vi "Send Request.vi"(8 "error in (no error)":errorcluster, 11 "MJPEG Reader in":refnum<class "MJPEG Reader.lvclass">) -> (0 "error out":errorcluster, 3 "MJPEG Reader out":refnum<class "MJPEG Reader.lvclass">)   [LabVIEW 2015, in "MJPEG Reader.lvclass"]
uses:
  MJPEG Reader.lvclass
  MJPEG Reader.lvclass/MJPEG Reader.ctl
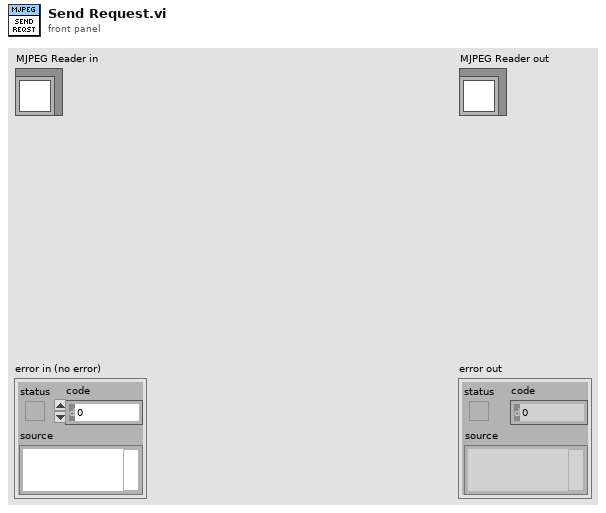
[diagram p1: front panel]
types:
  T1 = enum16{"Standard", "Buffered", "CRLF", "Immediate"}
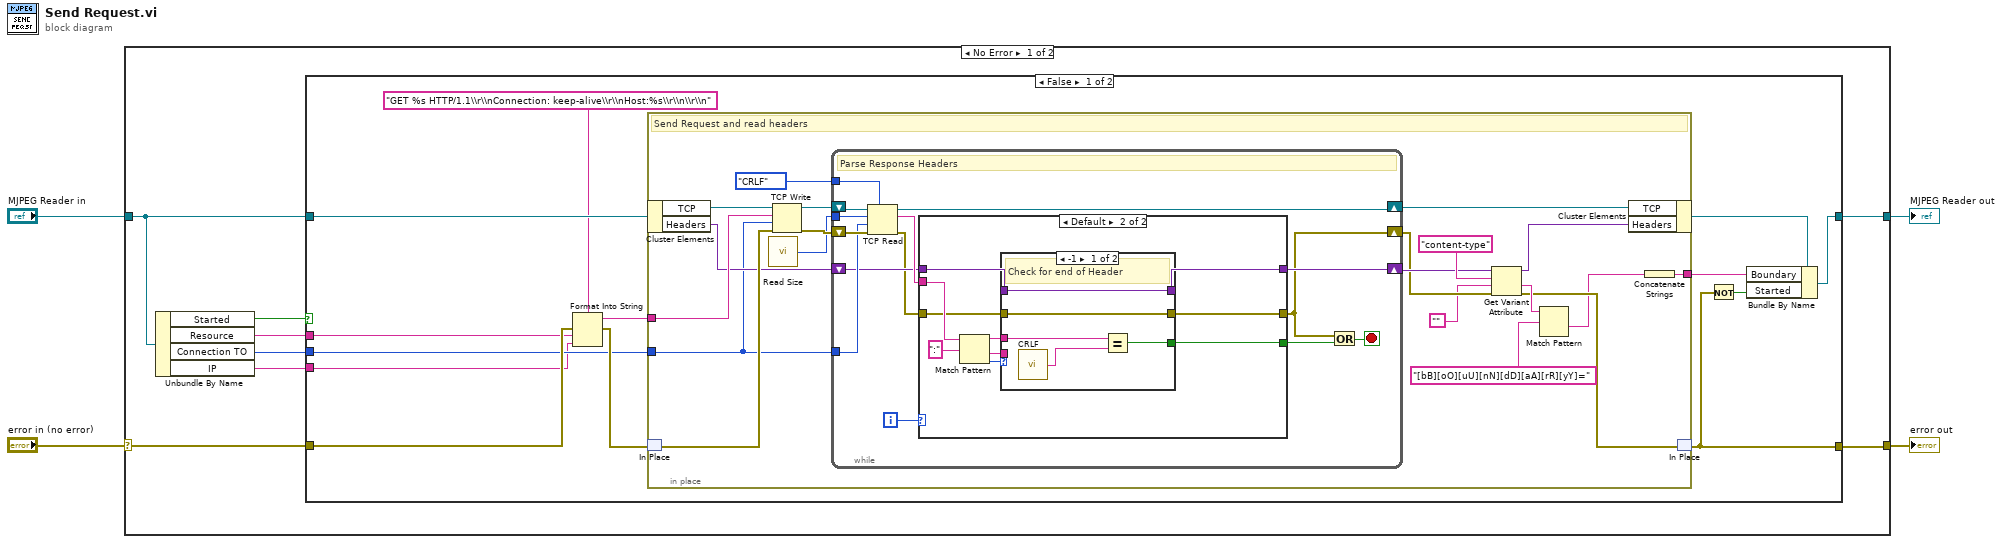
[diagram p0: block diagram]
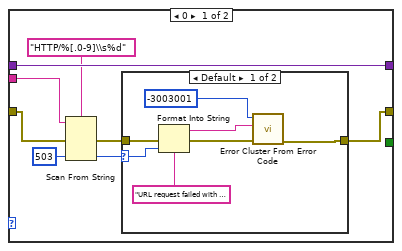
[diagram p2: hidden frame]
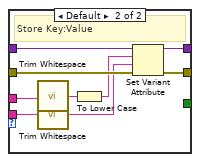
[diagram p4: hidden frame]
diagram:
  n1 = case shown="No Error" "error in (no error)" {
    selector: "error in (no error)" -> [w11 w103]
    tunnel: [w8 w103] -> w3
    tunnel: [w7 w102] -> w1
    tunnel: "MJPEG Reader in" -> [w12 w102]
    frame No Error {
      n2 = Unbundle By Name(w12) -> ("Started"=w6:bool, "Resource"=w10:string, "Connection TO"=w9:i32, "IP"=w5:string)
      n3 = case shown="False" w6 {
        tunnel: w12 -> [w25 w101]
        tunnel: w11 -> [w24 w100]
        tunnel: w10 -> [w22 _]
        tunnel: w9 -> [w19 _]
        tunnel: [w14 w100] -> w8
        tunnel: [w17 w101] -> w7
        tunnel: w5 -> [w13 _]
        frame False {
          n4 = Format Into String(format string="GET %s HTTP/1.1\\r\\nConnection: keep-alive\\r\\nHost:%s\\r\\n\\r\\n", error in=w24, w22, w13) -> (resulting string=w20:string, error out=w23:errorcluster)  [unwired: 1 in]
          n5 = in-place {
            in-place-border: w20 -> [w44]
            in-place-border: w19 -> [w36]
            in-place-border: [w26] -> w16
            # "Send Request and read headers"
            n6 = in-place-cluster #1(w25) -> ("TCP"=w45:refnum<k5>, "Headers"=w37:variant)
            n7 = in-place-match #2(w23) -> (w43:errorcluster)
            n8 = call "Read Size.vi"() -> ("bytes to read"=w39:i32)
            n9 = TCP Write(connection ID=w45, data in=w44, error in (no error)=w43, 9:w36) -> (connection ID out=w42:refnum<k5>, error out=w41:errorcluster)  [unwired: 1 out]
            n10 = while {
              shift-right: [w47] -> w33
              shift-left: w41 -> [w58]
              tunnel: T1."CRLF" ("mode (standard)") -> [w57]
              tunnel: w39 -> [w56]
              tunnel: w36 -> [w55]
              shift-right: [w53] -> w38
              shift-left: w42 -> [w59]
              shift-right: [w50] -> w34
              shift-left: w37 -> [w51]
              i -> [w46]
              stop <- w48 stop-if-true
              # "Parse Response Headers"
              n11 = TCP Read(connection ID=w59, bytes to read=w56, error in (no error)=w58, 7:w57, 9:w55) -> (connection ID out=w53:refnum<k5>, data out=w54:string, error out=w49:errorcluster)
              n12 = case shown="Default" w46 {
                tunnel: w54 -> [w63 w85]
                tunnel: [_ w81] -> w52
                tunnel: w51 -> [w67 w80]
                tunnel: [w67 w78] -> w50
                tunnel: w49 -> [w66 w77]
                tunnel: [w61 w76] -> w47
                frame 0 {
                  n13 = Scan From String(format string="HTTP/%[.0-9]\\s%d", input string=w63, error in=w66, default 2=503 ("default value 2")) -> (error out=w60:errorcluster, output 2=w62:i32)  [unwired: 3 in, 2 out]
                  n14 = case shown="Default" w62 {
                    selector: w62 -> [w73 _]
                    tunnel: [w68 w75] -> w61
                    tunnel: w60 -> [w74 w75]
                    frame Default {
                      n15 = Format Into String(format string="URL request failed with a code:%d.", error in=w74, w73) -> (resulting string=w70:string, error out=w71:errorcluster)  [unwired: 1 in]
                      n16 = call <vilib>:"Error Cluster From Error Code.vi"("error in (no error)"=w71, "error message (\"\")"=w70, "error code (0)"=-3003001) -> ("error out"=w68:errorcluster)  [unwired: 6 in]
                    }
                    frame 200 {
                    }
                  }
                }
                frame Default {
                  n17 = Match Pattern(string=w85, regular expression=":") -> (before substring=w82:string, after substring=w79:string, offset past match=w83:i32)  [unwired: 1 in, 1 out]
                  n18 = case shown="-1" w83 {
                    tunnel: w82 -> [w90 w99]
                    tunnel: [w89 _] -> w81
                    tunnel: w80 -> [w87 w96]
                    tunnel: w79 -> [_ w98]
                    tunnel: [w87 w95] -> w78
                    tunnel: w77 -> [w88 w94]
                    tunnel: [w88 w91] -> w76
                    frame -1 {
                      # "Check for end of Header"
                      n19 = call "CRLF.vi"() -> ("CRLF"=w86:string)
                      n20 = Equal?(x=w90, y=w86) -> (x = y?=w89:bool)
                    }
                    frame Default {
                      # "Store Key:Value"
                      n21 = call <vilib>:"Trim Whitespace.vi"("string"=w99) -> ("trimmed string"=w97:string)  [unwired: 1 in]
                      n22 = call <vilib>:"Trim Whitespace.vi"("string"=w98) -> ("trimmed string"=w92:string)  [unwired: 1 in]
                      n23 = To Lower Case(string=w97) -> (all lower case string=w93:string)
                      n24 = Set Variant Attribute(Variant=w96, name=w93, value=w92, error in=w94) -> (Variant out=w95:variant, error out=w91:errorcluster)  [unwired: 1 out]
                    }
                  }
                }
              }
              n25 = Or(x=w47, y=w52) -> (x .or. y?=w48:bool)
            }
            n26 = Get Variant Attribute(Variant=w34, name="content-type", default value (empty Variant)="", error in=w33) -> (duplicate Variant=w27:variant, value=w31:string, error out=w29:errorcluster)  [unwired: 1 out]
            n27 = Match Pattern(string=w31, regular expression="[bB][oO][uU][nN][dD][aA][rR][yY]=") -> (after substring=w28:string)  [unwired: 1 in, 3 out]
            n28 = in-place-cluster #1("TCP"=w38, "Headers"=w27) -> (w18:refnum<class "MJPEG Reader.lvclass">)
            n29 = Concatenate Strings(w28) -> (w26:string)
            n30 = in-place-match #2(w29) -> (w14:errorcluster)
          }
          n31 = Not(x=w14) -> (.not. x?=w15:bool)
          n32 = Bundle By Name(cluster=w18, "Boundary"=w16, "Started"=w15) -> (w17:refnum<class "MJPEG Reader.lvclass">)
        }
        frame True {
        }
      }
    }
    frame Error {
    }
  }
  "error out" <- w3
  "MJPEG Reader out" <- w1
